vi "Page_Info_Write.vi"(6 "ctlReferences":T1, 8 "error in (no error)":errorcluster, 10 "Target filename":string, 11 "AB_DepPackedLibrary in":refnum<class "AB_DepPackedLibrary.lvclass">) -> (0 "error out":errorcluster, 3 "AB_DepPackedLibrary out":refnum<class "AB_DepPackedLibrary.lvclass">)   [LabVIEW 2020, in "AB_DepPackedLibrary.lvclass"]
uses:
  <vilib>/AppBuilder/AB_Classes/DepPackedLib/AB_DepPackedLibrary.lvclass
  e:/builds/penguin/labview/branches/2020/dev/dist/vi.lib/AppBuilder/AB_Classes/Build/AB_Build.lvclass
  <resource>/Framework/Providers/Builds/AppBuilder/AB_UI_Page_Info_References.ctl
  <vilib>/AppBuilder/AB_Classes/PackedLib/AB_PackedLibrary.lvclass
  <vilib>/AppBuilder/AB_Classes/Deployment/AB_Deployment.lvlib
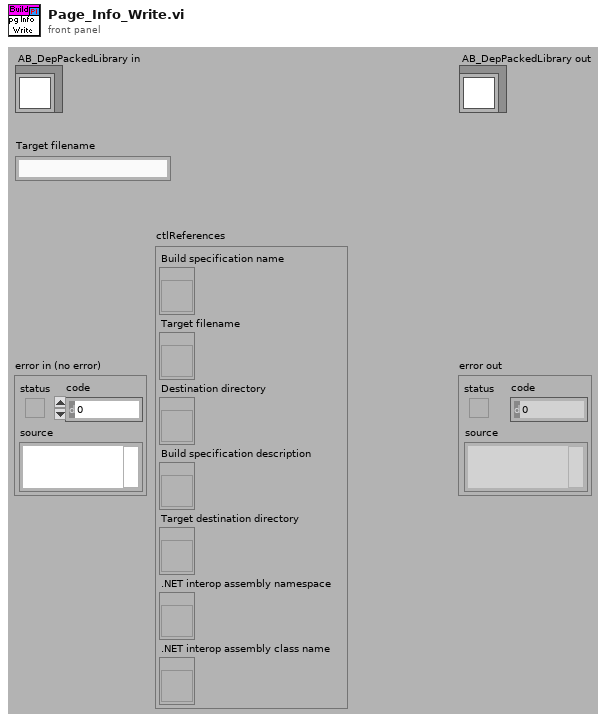
[diagram p1: front panel]
types:
  T1 = typedef "AB_UI_Page_Info_References.ctl" = cluster{"Build specification name":refnum<vi>, "Target filename":refnum<vi>, "Destination directory":refnum<vi>, "Build specification description":refnum<vi>, "Target destination directory":refnum<vi>, ".NET interop assembly namespace":refnum<vi>, ".NET interop assembly class name":refnum<vi>}
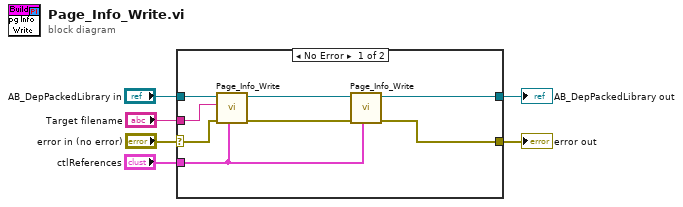
[diagram p0: block diagram]
diagram:
  n1 = case shown="No Error" "error in (no error)" {
    selector: "error in (no error)" -> [w8 w16]
    tunnel: [w10 w16] -> w2
    tunnel: [w11 w15] -> w1
    tunnel: "AB_DepPackedLibrary in" -> [w14 w15]
    tunnel: "ctlReferences" -> [w9 _]
    tunnel: "Target filename" -> [w13 _]
    frame No Error {
      n2 = call-parent <vilib>:"Page_Info_Write.vi"("ctlReferences"=w9, "error in (no error)"=w8, "Target filename"=w13, "AB_Targetfile in"=w14) -> ("error out"=w7:errorcluster, "AB_Targetfile out"=w12:refnum<class "AB_DepPackedLibrary.lvclass">)  [unwired: 6 in]
      n3 = call <vilib>:"Page_Info_Write.vi"("ctlReferences"=w9, "error in (no error)"=w7, "Build in"=w12) -> ("error out"=w10:errorcluster, "Build out"=w11:refnum<class "AB_DepPackedLibrary.lvclass">)  [unwired: 7 in]
    }
    frame Error {
    }
  }
  "error out" <- w2
  "AB_DepPackedLibrary out" <- w1
